vi "EventTouch_BallPossession.vi"(8 "Dist Para Toque":dbl=130.0, 9 "Tol para ang posse":dbl=0.3, 10 "Dist Para posse":dbl=180.0, 11 "IA State":T1={"our_robots"=[], "enemy_robots"=[], "balls"=[], "geometry"={"line_width"=0, "field_length"=0, "field_width"=0, "boundary_width"=0, "referee_width"=0, "goal_width"=0, "goal_depth"=0, "goal_wall_width"=0, "center_circle_radius"=0, "defense_radius"=0, "defense_stretch"=0, "free_kick_from_defense_dist"=0, "penalty_spot_from_field_line_dist"=0, "penalty_line_from_spot_dist"=0}, "IA Judge"={"stage"="", "command"="", "our_goalie_id"=0.0, "enemy_goalie_id"=0.0, "command enum"=enum."Halt", "Time"=enum."Azul"}, "Received Timestamp"=timestamp(0 s since 1904-01-01), "Events"={"Touch"=FALSE, "Ball out"=FALSE, "id touch"=0.0, "Ball out of \nVision"=FALSE, "Ball inside \nGoalie area"=FALSE, "Robot not responding"=FALSE, "Robots responding status"=[1.0, 1.0, 1.0, 1.0, 1.0, 1.0], "Enemy Ball \nPossession"=FALSE, "Pass State"=FALSE, "id end of pass"=0.0, "Kick"=FALSE, "Id ini Possession"=0.0, "Ball Possesion"=FALSE, "Id Possesion"=0.0}}) -> (0 "id touch":dbl, 1 "Toque":bool, 2 "id ini possesion":dbl, 3 "Posse inimigo":bool, 5 "id possesion":dbl, 7 "Posse nossa":bool)   [LabVIEW 2017]
uses:
  Core/AI Input.ctl
  Core/AI Robot.ctl
  Intel/Functions Enum.ctl
  Intel/AttackerStates.ctl
  Core/AI Ball.ctl
  Core/Field Size.ctl
  Core/AI Judge.ctl
  Intel/Command Enum.ctl
  Events.ctl
  <vilib>/Analysis/coordinate.llb/Wrap Angle (scalar).vi
  <vilib>/Analysis/NI_AAL_Angle.lvlib
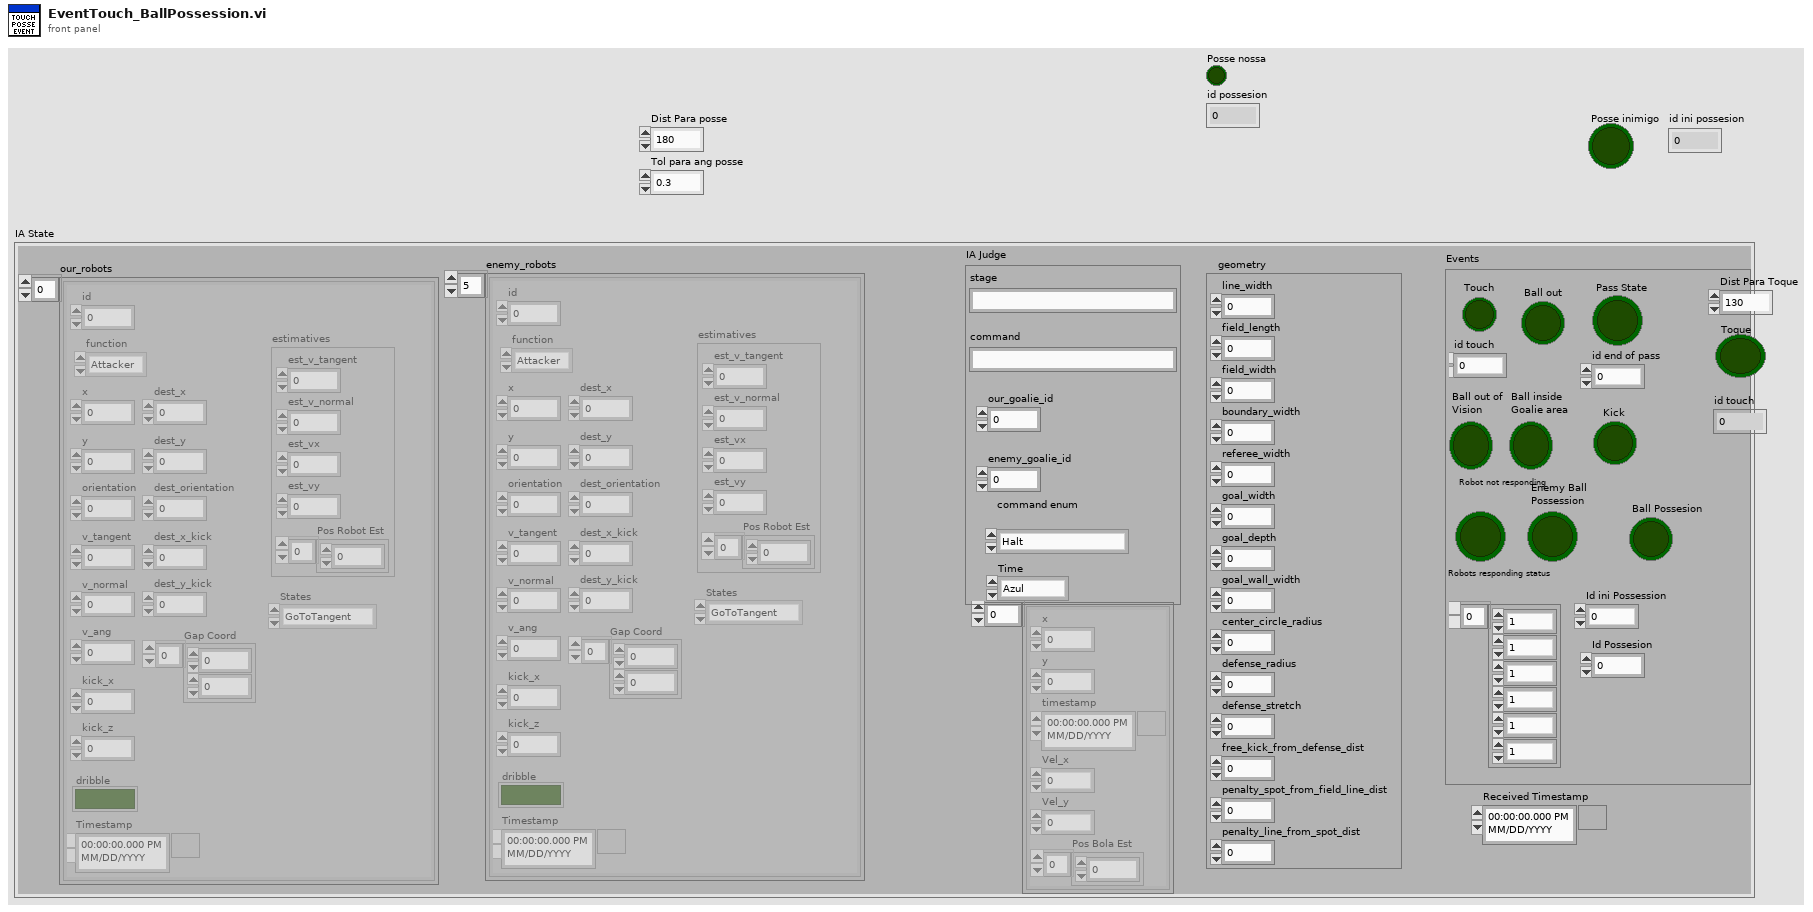
[diagram p1: front panel]
types:
  T1 = typedef "AI Input.ctl" = cluster{"our_robots":T2[], "enemy_robots":T2[], "balls":T5[], "geometry":T6, "IA Judge":T7, "Received Timestamp":timestamp, "Events":T9}
  T2 = typedef "AI Robot.ctl" = cluster{"id":u32, "function":T3, "x":dbl, "y":dbl, "orientation":dbl, "v_tangent":dbl, "v_normal":dbl, "v_ang":dbl, "kick_x":dbl, "kick_z":dbl, "dribble":bool, "Timestamp":timestamp, "dest_x":dbl, "dest_y":dbl, "dest_orientation":dbl, "estimatives":cluster{"est_v_tangent":dbl, "est_v_normal":dbl, "est_vx":dbl, "est_vy":dbl, "Pos Robot Est":dbl[]}, "dest_x_kick":dbl, "dest_y_kick":dbl, "Gap Coord":dbl[], "States":T4}
  T3 = typedef "Functions Enum.ctl" = enum16{"Attacker", "Goalie", "Defender", "Striker", "Goto 0", "Dummy", "Kicker", "ZigZag"}
  T4 = typedef "AttackerStates.ctl" = enum16{"Pass", "GoToTangent", "BallGetting", "GoToKick", ""}
  T5 = typedef "AI Ball.ctl" = cluster{"x":dbl, "y":dbl, "timestamp":timestamp, "Vel_x":dbl, "Vel_y":dbl, "Pos Bola Est":dbl[]}
  T6 = typedef "Field Size.ctl" = cluster{"line_width":u32, "field_length":u32, "field_width":u32, "boundary_width":u32, "referee_width":u32, "goal_width":u32, "goal_depth":u32, "goal_wall_width":u32, "center_circle_radius":u32, "defense_radius":u32, "defense_stretch":u32, "free_kick_from_defense_dist":u32, "penalty_spot_from_field_line_dist":u32, "penalty_line_from_spot_dist":u32}
  T7 = typedef "AI Judge.ctl" = cluster{"stage":string, "command":string, "our_goalie_id":dbl, "enemy_goalie_id":dbl, "command enum":T8, "Time":enum16{"Azul", "Amarelo"}}
  T8 = typedef "Command Enum.ctl" = enum16{"Halt", "Stop", "Force Start", "PKA Normal Start", "Prepare Kickoff Ally", "PKE Normal Start", "Prepare Kickoff Enemy", "Prepare Penalty Ally", "PPA Normal Start", "Prepare Penalty Enemy", "PPE Normal Start", "Direct Free Enemy", "Direct Free Ally", "Indirect Free Enemy", "Indirect Free Ally", "Timeout Enemy", "Timeout Ally", "Goal Enemy", "Goal Ally", "Ball Placement Enemy", "Ball Placement Ally", "Normal Half Time", "Extra Time Break", "Extra Half Time", "None", "Post Game"}
  T9 = typedef "Events.ctl" = cluster{"Touch":bool, "Ball out":bool, "id touch":dbl, "Ball out of \nVision":bool, "Ball inside \nGoalie area":bool, "Robot not responding":bool, "Robots responding status":dbl[], "Enemy Ball \nPossession":bool, "Pass State":bool, "id end of pass":dbl, "Kick":bool, "Id ini Possession":dbl, "Ball Possesion":bool, "Id Possesion":dbl}
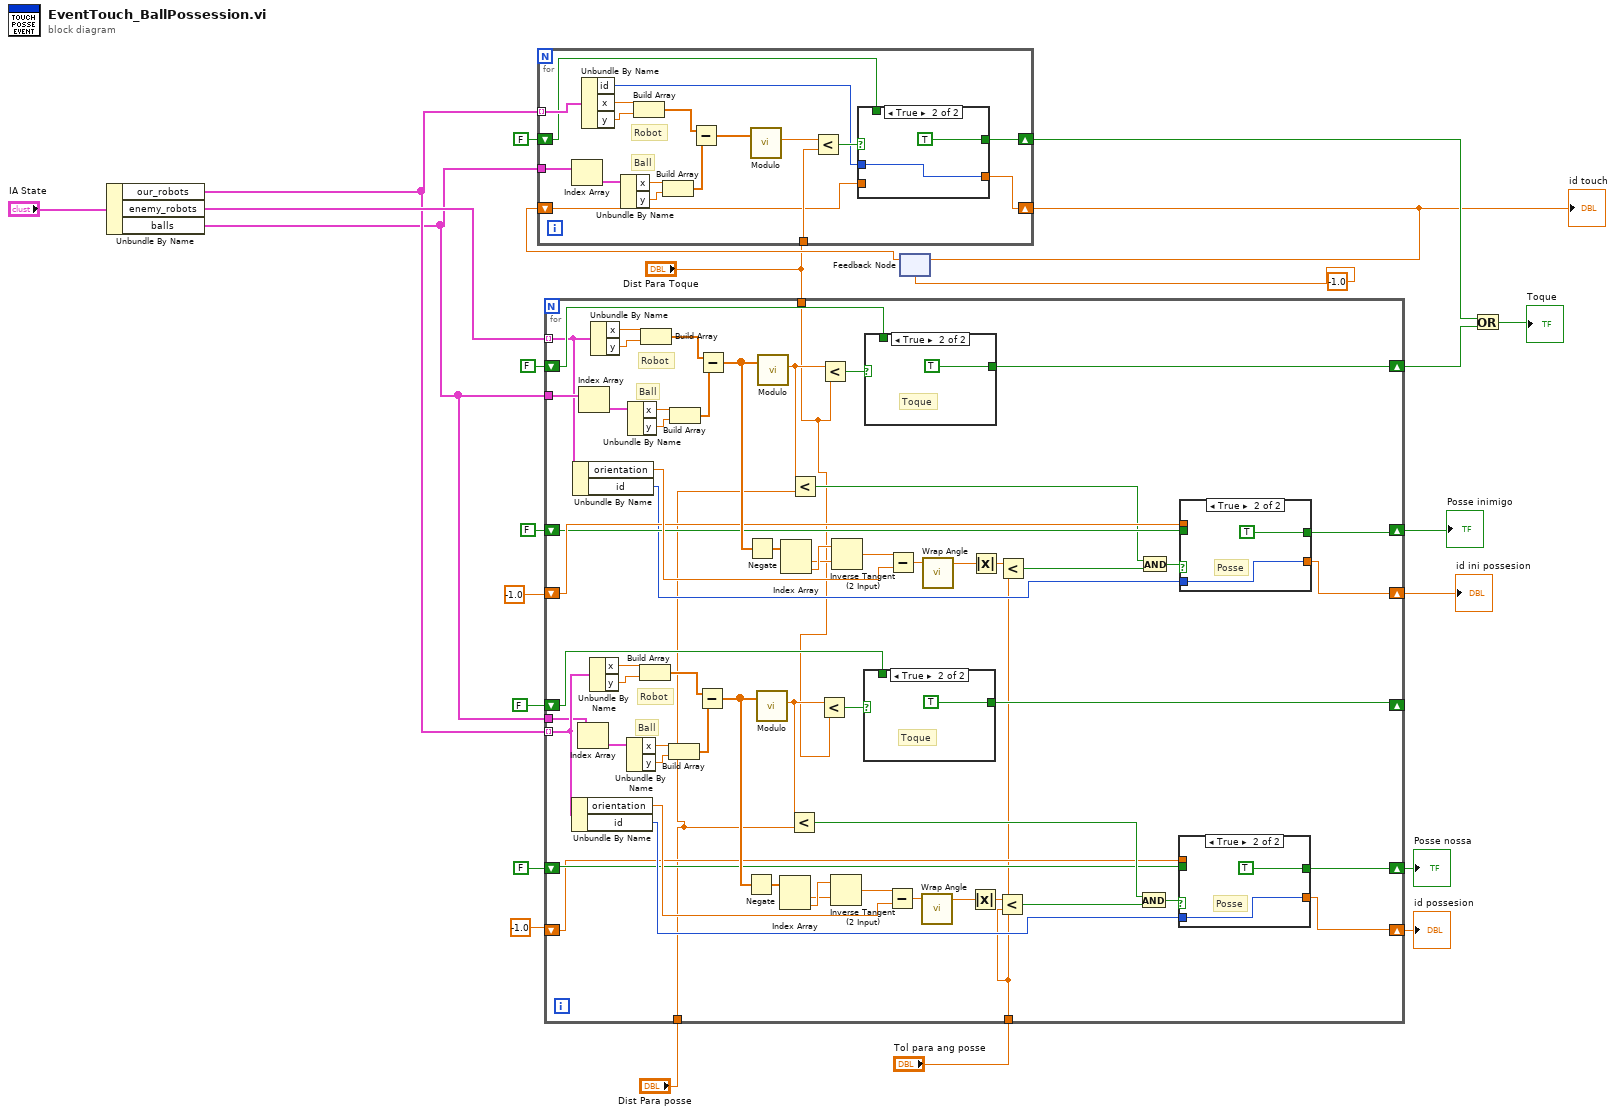
[diagram p0: block diagram]
diagram:
  n1 = Unbundle By Name("IA State") -> ("our_robots"=w4:T2[], "enemy_robots"=w20:T2[], "balls"=w3:T5[])
  n2 = for {
    tunnel: w20 -> [w76] mode=indexing
    tunnel: w3 -> [w87]
    shift-right: [w78] -> w19
    shift-left: FALSE -> [w77]
    tunnel: "Dist Para Toque" -> [w27]
    tunnel: "Tol para ang posse" -> [w25]
    shift-right: [w59] -> w8
    shift-left: -1.0 -> [w64]
    tunnel: "Dist Para posse" -> [w26]
    shift-right: [w63] -> w9
    shift-left: FALSE -> [w62]
    shift-right: [w34] -> _
    shift-left: FALSE -> [w35]
    shift-right: [w30] -> w2
    shift-left: FALSE -> [w33]
    shift-right: [w31] -> w1
    shift-left: -1.0 -> [w32]
    tunnel: w4 -> [w29] mode=indexing
    tunnel: w3 -> [w28]
    # "Ball"
    # "Robot"
    # "Ball"
    # "Robot"
    n3 = Unbundle By Name(w29) -> ("orientation"=w41:dbl, "id"=w36:u32)
    n4 = Unbundle By Name(w76) -> ("orientation"=w67:dbl, "id"=w58:u32)
    n5 = Index Array(array=w28) -> (element=w57:T5)  [unwired: 1 in]
    n6 = Index Array(array=w87) -> (element=w86:T5)  [unwired: 1 in]
    n7 = Unbundle By Name(w29) -> ("x"=w54:dbl, "y"=w53:dbl)
    n8 = Unbundle By Name(w76) -> ("x"=w83:dbl, "y"=w82:dbl)
    n9 = Unbundle By Name(w57) -> ("x"=w56:dbl, "y"=w55:dbl)
    n10 = Unbundle By Name(w86) -> ("x"=w85:dbl, "y"=w84:dbl)
    n11 = Build Array(w54, w53) -> (w52:dbl[])
    n12 = Build Array(w83, w82) -> (w81:dbl[])
    n13 = Build Array(w56, w55) -> (w51:dbl[])
    n14 = Build Array(w85, w84) -> (w80:dbl[])
    n15 = Subtract(x=w52, y=w51) -> (x-y=w42:dbl[])
    n16 = Subtract(x=w81, y=w80) -> (x-y=w68:dbl[])
    n17 = Negate(x=w42) -> (-x=w49:dbl[])
    n18 = Negate(x=w68) -> (-x=w75:dbl[])
    n19 = call "Modulo.vi"("2D vector"=w42) -> ("Modulo"=w40:dbl)  [unwired: 10 in]
    n20 = call "Modulo.vi"("2D vector"=w68) -> ("Modulo"=w66:dbl)  [unwired: 10 in]
    n21 = Index Array(array=w49) -> (element #1=w47:dbl, element #2=w48:dbl)  [unwired: 2 in]
    n22 = Index Array(array=w75) -> (element #1=w73:dbl, element #2=w74:dbl)  [unwired: 2 in]
    n23 = Less?(x=w40, y=w26) -> (x < y?=w37:bool)
    n24 = Less?(x=w66, y=w26) -> (x < y?=w60:bool)
    n25 = Less?(x=w40, y=w27) -> (x < y?=w50:bool)
    n26 = Less?(x=w66, y=w27) -> (x < y?=w79:bool)
    n27 = Inverse Tangent (2 Input)(1:w47, 2:w48) -> (0:w46:dbl)
    n28 = Inverse Tangent (2 Input)(1:w73, 2:w74) -> (0:w72:dbl)
    n29 = case shown="True" w50 {
      tunnel: [w92 TRUE] -> w34
      tunnel: w35 -> [w92 _]
      frame False {
        # "Sem toque"
      }
      frame True {
        # "Toque"
      }
    }
    n30 = case shown="True" w79 {
      tunnel: [w98 TRUE] -> w78
      tunnel: w77 -> [w98 _]
      frame False {
        # "Sem toque"
      }
      frame True {
        # "Toque"
      }
    }
    n31 = Subtract(x=w46, y=w41) -> (x-y=w45:dbl)
    n32 = Subtract(x=w72, y=w67) -> (x-y=w71:dbl)
    n33 = call-poly <vilib>:"Wrap Angle.vi"("angle in"=w45) -> ("angle out"=w43:dbl)  [unwired: 9 in, 1 out]
    n34 = call-poly <vilib>:"Wrap Angle.vi"("angle in"=w71) -> ("angle out"=w69:dbl)  [unwired: 9 in, 1 out]
    n35 = Absolute Value(x=w43) -> (abs(x)=w44:dbl)
    n36 = Absolute Value(x=w69) -> (abs(x)=w70:dbl)
    n37 = Less?(x=w44, y=w25) -> (x < y?=w38:bool)
    n38 = Less?(x=w70, y=w25) -> (x < y?=w61:bool)
    n39 = And(x=w37, y=w38) -> (x .and. y?=w39:bool)
    n40 = And(x=w60, y=w61) -> (x .and. y?=w65:bool)
    n41 = case shown="True" w39 {
      tunnel: [w88 TRUE] -> w30
      tunnel: w36 -> [_ w90]
      tunnel: [w89 w90] -> w31
      tunnel: w32 -> [w89 _]
      tunnel: w33 -> [w88 _]
      frame False {
        # "Sem toque"
      }
      frame True {
        # "Posse"
      }
    }
    n42 = case shown="True" w65 {
      tunnel: [w94 TRUE] -> w63
      tunnel: w58 -> [_ w96]
      tunnel: [w95 w96] -> w59
      tunnel: w64 -> [w95 _]
      tunnel: w62 -> [w94 _]
      frame False {
        # "Sem toque"
      }
      frame True {
        # "Posse"
      }
    }
  }
  "Posse inimigo" <- w9
  "id ini possesion" <- w8
  "Posse nossa" <- w2
  "id possesion" <- w1
  n43 = feedback #1(-1.0) -> (w16:dbl)
  n44 = for {
    tunnel: w4 -> [w113] mode=indexing
    tunnel: w3 -> [w117]
    shift-right: [w105] -> w22
    shift-left: FALSE -> [w104]
    tunnel: "Dist Para Toque" -> [w103]
    shift-right: [w102] -> w17
    shift-left: w16 -> [w100]
    # "Ball"
    # "Robot"
    n45 = Index Array(array=w117) -> (element=w116:T5)  [unwired: 1 in]
    n46 = Unbundle By Name(w113) -> ("id"=w101:u32, "x"=w112:dbl, "y"=w111:dbl)
    n47 = Unbundle By Name(w116) -> ("x"=w115:dbl, "y"=w114:dbl)
    n48 = Build Array(w112, w111) -> (w110:dbl[])
    n49 = Build Array(w115, w114) -> (w109:dbl[])
    n50 = Subtract(x=w110, y=w109) -> (x-y=w108:dbl[])
    n51 = call "Modulo.vi"("2D vector"=w108) -> ("Modulo"=w106:dbl)  [unwired: 10 in]
    n52 = Less?(x=w106, y=w103) -> (x < y?=w107:bool)
    n53 = case shown="True" w107 {
      tunnel: [w119 TRUE] -> w105
      tunnel: w104 -> [w119 _]
      tunnel: [w118 w120] -> w102
      tunnel: w101 -> [_ w120]
      tunnel: w100 -> [w118 _]
      frame False {
      }
      frame True {
      }
    }
  }
  "id touch" <- w17
  n54 = feedback-in #1(w17) -> ()
  n55 = Or(x=w22, y=w19) -> (x .or. y?=→"Toque":bool)
